vi "trapezoidal.vi"(6 "Ciclos":dbl, 7 "%Subida":dbl, 8 "Frequencia":dbl, 9 "Amplitude":dbl, 10 "%Descida":dbl, 11 "%Alto":dbl) -> (3 "Waveform Graph":waveform(dbl)(graph))   [LabVIEW 2018]
uses:
  <vilib>/Analysis/1siggen.llb/Ramp Pattern by Samples.vi
  <vilib>/Analysis/NI_AALBase.lvlib
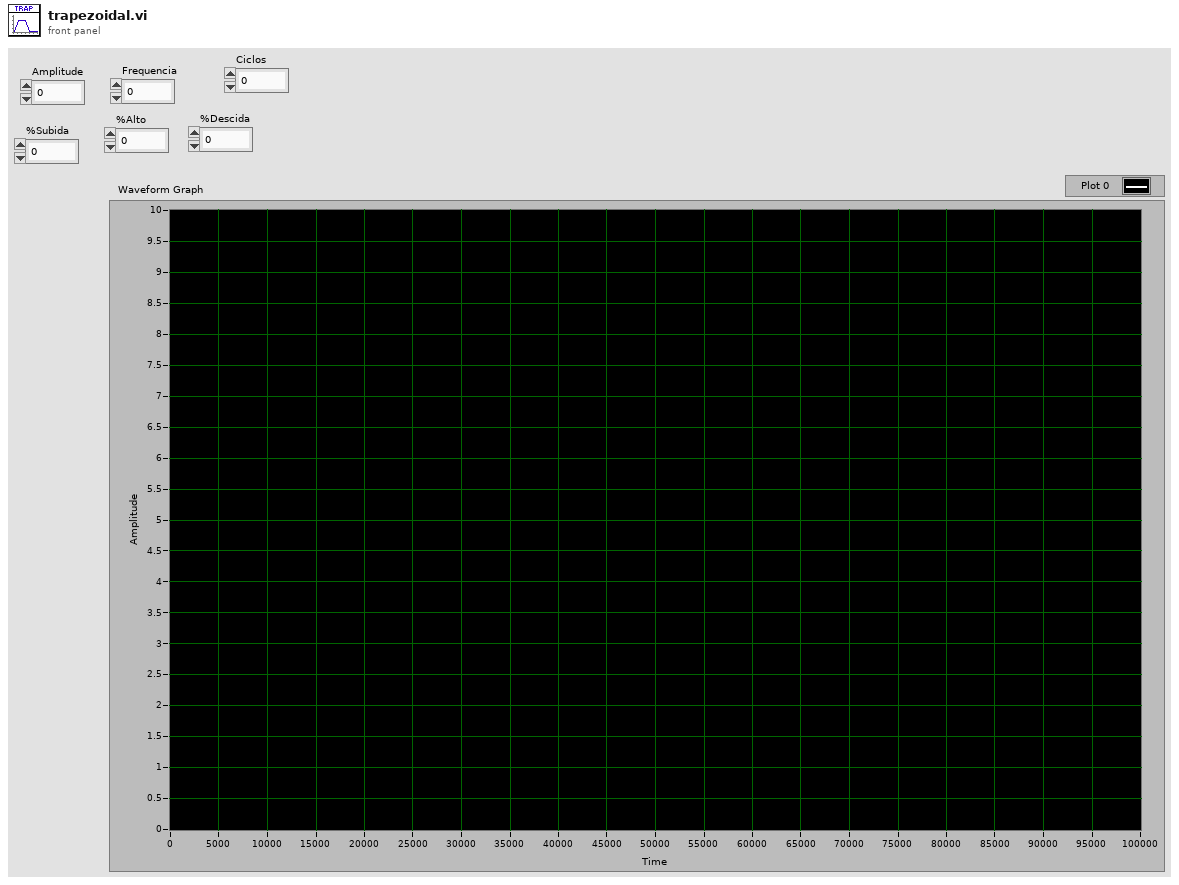
[diagram p1: front panel]
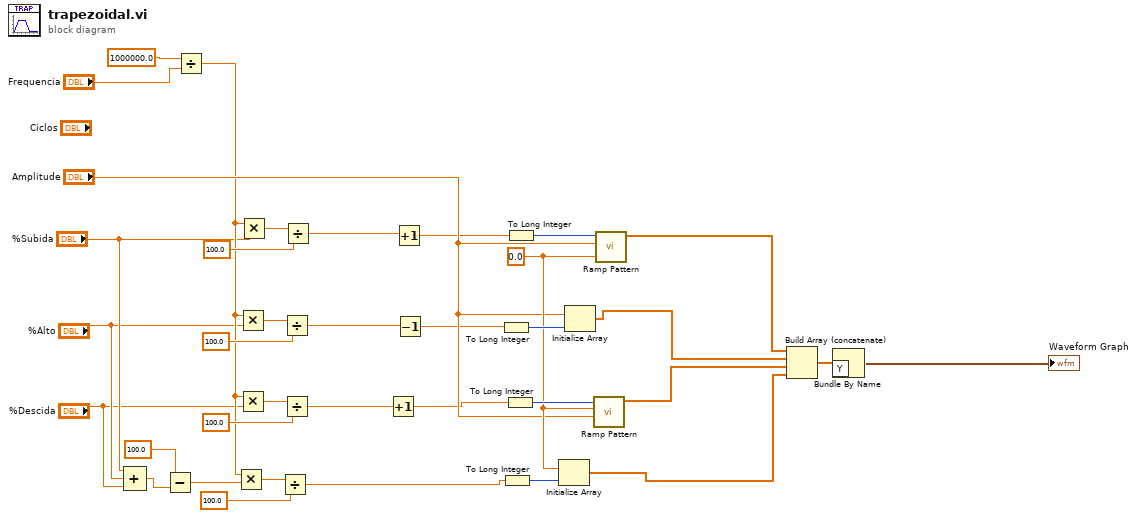
[diagram p0: block diagram]
diagram:
  w28 = 0.0 ("start")
  n1 = Compound Arithmetic op=ADD("%Subida", "%Alto", "%Descida") -> (w4:dbl)
  n2 = Subtract(x=100.0, y=w4) -> (x-y=w2:dbl)
  n3 = Divide(x=1000000.0, y="Frequencia") -> (x/y=w11:dbl)
  n4 = Multiply(x=w11, y=w2) -> (x*y=w13:dbl)
  n5 = Multiply(x=w11, y="%Alto") -> (x*y=w17:dbl)
  n6 = Multiply(x=w11, y="%Descida") -> (x*y=w15:dbl)
  n7 = Multiply(x=w11, y="%Subida") -> (x*y=w20:dbl)
  n8 = Divide(x=w13, y=100.0) -> (x/y=w8:dbl)
  n9 = Divide(x=w17, y=100.0) -> (x/y=w10:dbl)
  n10 = Divide(x=w15, y=100.0) -> (x/y=w9:dbl)
  n11 = Divide(x=w20, y=100.0) -> (x/y=w18:dbl)
  n12 = Increment(x=w9) -> (x+1=w24:dbl)
  n13 = Increment(x=w18) -> (x+1=w26:dbl)
  n14 = Decrement(x=w10) -> (x-1=w25:dbl)
  n15 = To Long Integer(number=w25) -> (32bit integer=w32:i32)
  n16 = To Long Integer(number=w8) -> (32bit integer=w30:i32)
  n17 = To Long Integer(number=w24) -> (32bit integer=w35:i32)
  n18 = To Long Integer(number=w26) -> (32bit integer=w36:i32)
  n19 = Initialize Array(w28, w30) -> (w29:dbl[])
  n20 = Initialize Array("Amplitude", w32) -> (w31:dbl[])
  n21 = call-poly <vilib>:"Ramp Pattern.vi"("start"="Amplitude", "end"=w28, "samples"=w35) -> ("Ramp Pattern"=w33:dbl[])  [unwired: 7 in, 1 out]
  n22 = call-poly <vilib>:"Ramp Pattern.vi"("start"=w28, "end"="Amplitude", "samples"=w36) -> ("Ramp Pattern"=w34:dbl[])  [unwired: 7 in, 1 out]
  n23 = Build Array (concatenate)(w34, w31, w33, w29) -> (w23:dbl[])
  n24 = Bundle By Name("Y"=w23) -> (→"Waveform Graph":waveform(dbl))  [unwired: 1 in]
